vi "TPNT_AlarmActions.vi"(2 "tpnt_logfile":path, 3 "mailserver":string="localhost", 4 "tpnt type":string, 5 "action":enum16{"send", "clear", "clear all"}(ring), 6 "curr val":string, 7 "TP name":string, 8 "error in (no error)":errorcluster, 9 "device":string, 10 "alarm field":string, 11 "alarm message":string) -> (0 "error out":errorcluster)   [LabVIEW 2016]
panel:
  in  "AlarmsArray":T1(array[cluster])
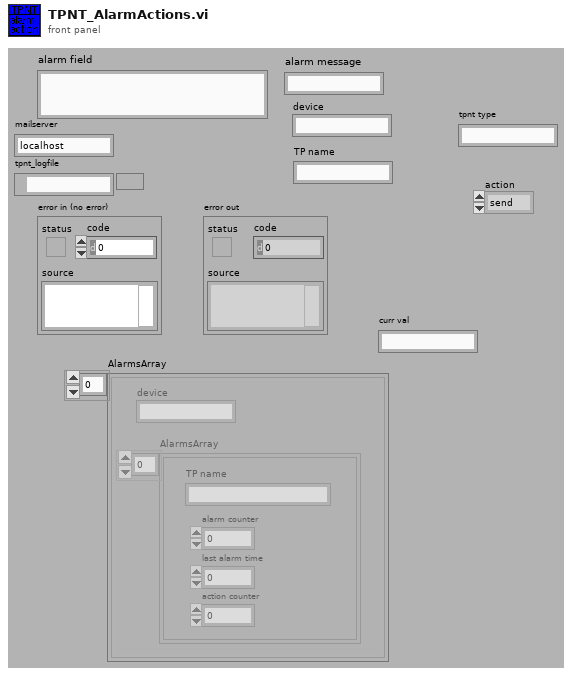
[diagram p1: front panel]
types:
  T1 = cluster{"device":string, "AlarmsArray":cluster{"TP name":string, "alarm counter":i32, "last alarm time":u32, "action counter":i32}[]}[]
  T2 = cluster{"device":string, cluster{"TP name":string, i32, i32, i32}[]}
  T3 = cluster{"device":string, "AlarmsArray":cluster{"TP name":string, "alarm counter":i32, "last alarm time":u32, "action counter":i32}[]}
  T4 = cluster{"TP name":string, "alarm counter":i32, "last alarm time":u32, "action counter":i32}[]
  T5 = cluster{"TP name":string, i32, "millisecond timer value":u32, i32}
  T6 = cluster{"TP name":string, "alarm counter":i32, "last alarm time":u32, "action counter":i32}
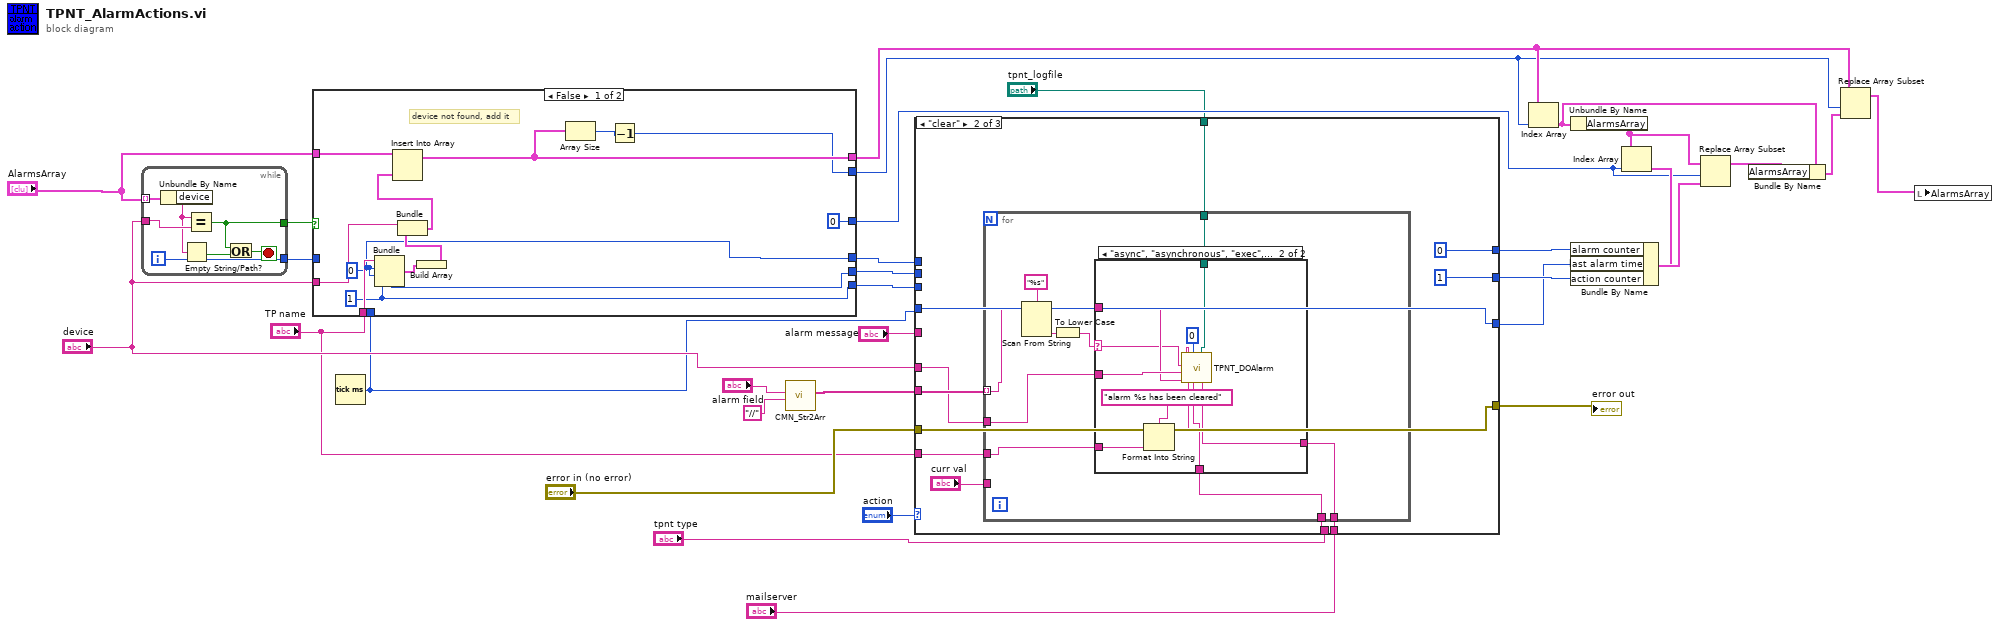
[diagram p0: block diagram]
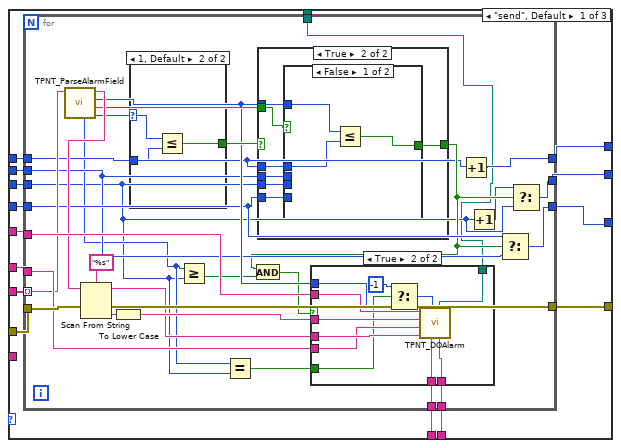
[diagram p2: hidden frame]
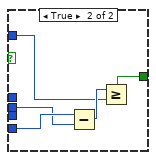
[diagram p5: hidden frame]
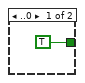
[diagram p6: hidden frame]
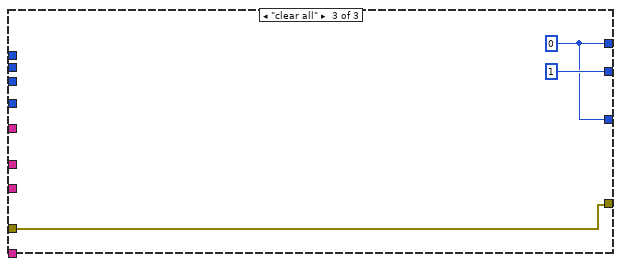
[diagram p8: hidden frame]
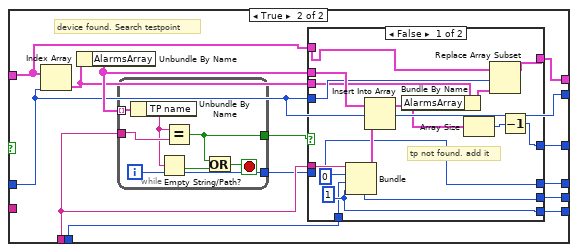
[diagram p9: hidden frame]
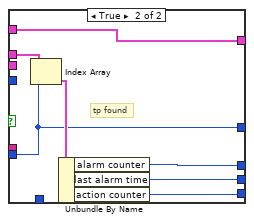
[diagram p10: hidden frame]
diagram:
  n1 = while {
    tunnel: "AlarmsArray" -> [w39] mode=indexing
    tunnel: "device" -> [w38]
    tunnel: [w34] -> w26
    tunnel: [w33] -> w25
    i -> [w33]
    stop <- w35 stop-if-true
    n2 = Unbundle By Name(w39) -> ("device"=w36:string)
    n3 = Empty String/Path?(string/path=w36) -> (empty?=w37:bool)
    n4 = Equal?(x=w36, y=w38) -> (x = y?=w34:bool)
    n5 = Or(x=w34, y=w37) -> (x .or. y?=w35:bool)
  }
  n6 = Tick Count (ms)() -> (millisecond timer value=w5:u32)
  n7 = case shown="False" w26 {
    tunnel: w25 -> [_ w54]
    tunnel: "AlarmsArray" -> [w51 w59]
    tunnel: "TP name" -> [w48 w63]
    tunnel: "device" -> [w50 _]
    tunnel: [w40 w61] -> w12
    tunnel: [w44 w58] -> w15
    tunnel: [w40 w56] -> w11
    tunnel: [w45 w55] -> w10
    tunnel: [w42 w54] -> w14
    tunnel: [0 w53] -> w19
    tunnel: w5 -> [_ w52]
    frame False {
      w45 = 1
      w40 = 0
      # "device not found, add it"
      n8 = Bundle("TP name"=w48, w40, w40, w45) -> (w49:cluster{"TP name":string, i32, i32, i32})  [unwired: 1 out]
      n9 = Build Array(w49) -> (w47:cluster{"TP name":string, i32, i32, i32}[])
      n10 = Bundle("device"=w50, w47) -> (w46:T2)  [unwired: 1 out]
      n11 = Insert Into Array(array=w51, new element=w46) -> (w44:T1)  [unwired: 1 in]
      n12 = Array Size(array=w44) -> (size(s)=w43:i32)
      n13 = Decrement(x=w43) -> (x-1=w42:i32)
    }
    frame True {
      # "device found. Search testpoint"
      n14 = Index Array(array=w59, index=w54) -> (element=w57:T3)
      n15 = Unbundle By Name(w57) -> ("AlarmsArray"=w62:T4)
      n16 = while {
        tunnel: w62 -> [w92] mode=indexing
        tunnel: w63 -> [w91]
        tunnel: [w87] -> w64
        tunnel: [w86] -> w60
        i -> [w86]
        stop <- w88 stop-if-true
        n17 = Unbundle By Name(w92) -> ("TP name"=w89:string)
        n18 = Empty String/Path?(string/path=w89) -> (empty?=w90:bool)
        n19 = Equal?(x=w89, y=w91) -> (x = y?=w87:bool)
        n20 = Or(x=w87, y=w90) -> (x .or. y?=w88:bool)
      }
      n21 = case shown="False" w64 {
        tunnel: [w70 w83] -> w61
        tunnel: w63 -> [w77 _]
        tunnel: w62 -> [w76 w85]
        tunnel: w60 -> [_ w79]
        tunnel: w59 -> [w75 w82]
        tunnel: [w74 w82] -> w58
        tunnel: w54 -> [w73 _]
        tunnel: w57 -> [w72 _]
        tunnel: [w65 w81] -> w56
        tunnel: [w69 w80] -> w55
        tunnel: [w66 w79] -> w53
        tunnel: w52 -> [w65 _]
        frame False {
          w69 = 1
          w70 = 0
          # "tp not found. add it"
          n22 = Bundle("TP name"=w77, w70, "millisecond timer value"=w65, w69) -> (w78:T5)  [unwired: 1 out]
          n23 = Insert Into Array(array=w76, new element=w78) -> (w68:T4)  [unwired: 1 in]
          n24 = Bundle By Name(cluster=w72, "AlarmsArray"=w68) -> (w71:T3)
          n25 = Array Size(array=w68) -> (size(s)=w67:i32)
          n26 = Replace Array Subset(array=w75, new element=w71, index=w73) -> (w74:T1)
          n27 = Decrement(x=w67) -> (x-1=w66:i32)
        }
        frame True {
          # "tp found"
          n28 = Index Array(array=w85, index=w79) -> (element=w84:T6)
          n29 = Unbundle By Name(w84) -> ("alarm counter"=w83:i32, "last alarm time"=w81:u32, "action counter"=w80:i32)
        }
      }
    }
  }
  n30 = call "CMN_Str2Arr.vi"("separator"="//", "string in"="alarm field") -> ("Array out"=w27:string[])  [unwired: 2 in, 7 out]
  n31 = case shown="\"clear\"" "action" {
    tunnel: "alarm message" -> [w107 _ _]
    tunnel: "error in (no error)" -> [w106 w177 w201]
    tunnel: w27 -> [w105 w175 _]
    tunnel: "device" -> [w104 w174 _]
    tunnel: [w103 w177 w201] -> w23
    tunnel: w12 -> [w102 _ _]
    tunnel: w11 -> [w101 _ _]
    tunnel: w10 -> [w100 _ _]
    tunnel: [w99 0 w200] -> w9
    tunnel: [w98 1 1] -> w8
    tunnel: [w96 w176 w200] -> w6
    tunnel: w5 -> [w97 w176 _]
    tunnel: "TP name" -> [_ w173 _]
    tunnel: "tpnt type" -> [w95 w170 _]
    tunnel: "mailserver" -> [w94 w171 _]
    tunnel: "tpnt_logfile" -> [w93 w169 _]
    frame "send", Default {
      n32 = for {
        tunnel: w104 -> [w126]
        tunnel: w107 -> [w132]
        tunnel: w106 -> [w136]
        tunnel: w105 -> [w125] mode=indexing
        tunnel: [w133] -> w103
        tunnel: w102 -> [w114]
        tunnel: w101 -> [w119]
        tunnel: w100 -> [w112]
        tunnel: [w123] -> w99
        tunnel: [w122] -> w98
        tunnel: w97 -> [w121]
        tunnel: [w120] -> w96
        tunnel: w95 -> [w110]
        tunnel: w94 -> [w109]
        tunnel: w93 -> [w108]
        n33 = call "TPNT_ParseAlarmField.vi"("Alarm Field"=w125) -> ("after"=w129:i32, "every msecs"=w128:bool, "every"=w124:i32, "action"=w130:string, "max"=w113:i32)  [unwired: 1 in, 5 out]
        n34 = Scan From String(format string="%s", input string=w130, error in=w136) -> (remaining string=w127:string, error out=w133:errorcluster, output 1=w135:string)  [unwired: 1 in, 2 out]
        n35 = To Lower Case(string=w135) -> (all lower case string=w131:string)
        n36 = case shown="1, Default" w129 {
          selector: w129 -> [_ w168]
          tunnel: w114 -> [_ w167]
          tunnel: [TRUE w166] -> w134
          frame ..0 {
          }
          frame 1, Default {
            n37 = Less Or Equal?(x=w168, y=w167) -> (x <= y?=w166:bool)
          }
        }
        n38 = Greater Or Equal?(x=w113, y=w112) -> (x >= y?=w117:bool)
        n39 = Equal?(x=w113, y=w112) -> (x = y?=w111:bool)
        n40 = case shown="True" w134 {
          selector: w134 -> [w149 _]
          tunnel: w124 -> [_ w153]
          tunnel: w119 -> [_ w156]
          tunnel: [w149 w155] -> w118
          tunnel: w112 -> [_ w154]
          tunnel: w128 -> [_ w152]
          tunnel: w121 -> [_ w151]
          tunnel: w114 -> [_ w150]
          frame False {
          }
          frame True {
            n41 = case shown="False" w152 {
              tunnel: w156 -> [_ w162]
              tunnel: [w159 w164] -> w155
              tunnel: w154 -> [_ _]
              tunnel: w153 -> [w158 w160]
              tunnel: w151 -> [_ w163]
              tunnel: w150 -> [w157 _]
              frame False {
                n42 = Less Or Equal?(x=w158, y=w157) -> (x <= y?=w159:bool)
              }
              frame True {
                n43 = Subtract(x=w163, y=w162) -> (x-y=w161:u32)
                n44 = Greater Or Equal?(x=w161, y=w160) -> (x >= y?=w164:bool)
              }
            }
          }
        }
        n45 = And(x=w118, y=w117) -> (x .and. y?=w116:bool)
        n46 = case shown="True" w116 {
          tunnel: w132 -> [_ w148]
          tunnel: w131 -> [_ w147]
          tunnel: w127 -> [_ w146]
          tunnel: w126 -> [_ w145]
          tunnel: w124 -> [_ w143]
          tunnel: w111 -> [_ w144]
          tunnel: w110 -> [_ w140]
          tunnel: w109 -> [_ w139]
          tunnel: w108 -> [_ w138]
          frame False {
          }
          frame True {
            n47 = Select(t=-1, s=w144, f=w143) -> (s? t:f=w141:i32)
            n48 = call "TPNT_DOAlarm.vi"("mailserver"=w139, "tpnt_logfile"=w138, "tpnt type"=w140, "next alarm (msecs)"=w141, "arguments"=w146, "device"=w145, "action"=w147, "alarm message"=w148) -> ()  [unwired: 4 out]
          }
        }
        n49 = Increment(x=w114) -> (x+1=w123:i32)
        n50 = Increment(x=w112) -> (x+1=w115:i32)
        n51 = Select(t=w121, s=w118, f=w119) -> (s? t:f=w120:u32)
        n52 = Select(t=w115, s=w118, f=w112) -> (s? t:f=w122:i32)
      }
    }
    frame "clear" {
      n53 = for {
        tunnel: w175 -> [w185] mode=indexing
        tunnel: w174 -> [w187]
        tunnel: w173 -> [w181]
        tunnel: "curr val" -> [_]
        tunnel: w171 -> [w189]
        tunnel: w170 -> [w188]
        tunnel: w169 -> [w180]
        n54 = Scan From String(format string="%s", input string=w185) -> (remaining string=w183:string, output 1=w186:string)  [unwired: 2 in, 3 out]
        n55 = To Lower Case(string=w186) -> (all lower case string=w182:string)
        n56 = case shown="\"async\", \"asynchronous\", \"exec\", \"mail\", \"mailto\", \"script\", \"sysexec\", \"umail\", \"umailto\"" w182 {
          selector: w182 -> [_ w194]
          tunnel: w189 -> [_ w198]
          tunnel: w188 -> [_ w197]
          tunnel: w187 -> [_ w196]
          tunnel: w183 -> [_ w195]
          tunnel: w181 -> [_ w192]
          tunnel: w180 -> [_ w190]
          frame Default {
          }
          frame "async", "asynchronous", "exec", "mail", "mailto", "script", "sysexec", "umail", "umailto" {
            n57 = Format Into String(format string="alarm %s has been cleared" ("alarm message"), w192) -> (resulting string=w191:string)  [unwired: 2 in, 1 out]
            n58 = call "TPNT_DOAlarm.vi"("mailserver"=w198, "tpnt_logfile"=w190, "tpnt type"=w197, "next alarm (msecs)"=0, "arguments"=w195, "device"=w196, "action"=w194, "alarm message"=w191) -> ()  [unwired: 4 out]
          }
        }
      }
    }
    frame "clear all" {
      w200 = 0
    }
  }
  "error out" <- w23
  n59 = Index Array(array=w15, index=w14) -> (element=w17:T3)
  n60 = Unbundle By Name(w17) -> ("AlarmsArray"=w20:T4)
  n61 = Index Array(array=w20, index=w19) -> (element=w21:T6)
  n62 = Bundle By Name(cluster=w21, "alarm counter"=w9, "last alarm time"=w6, "action counter"=w8) -> (w22:T6)
  n63 = Replace Array Subset(array=w20, new element=w22, index=w19) -> (w18:T4)
  n64 = Bundle By Name(cluster=w17, "AlarmsArray"=w18) -> (w16:T3)
  n65 = Replace Array Subset(array=w15, new element=w16, index=w14) -> (w13:T1)
  n66 = local write "AlarmsArray"(w13) -> ()
